vi "Do.vi"(8 "error in (no error)":errorcluster, 10 "Actor in":refnum<class "Actor.lvclass">, 11 "tt20panel_connect Msg":refnum<class "tt20panel_connect Msg.lvclass">) -> (0 "error out":errorcluster, 2 "Actor out":refnum<class "Actor.lvclass">)   [LabVIEW 2015, in "tt20panel_connect Msg.lvclass"]
doc: "This VI delivers the message to the actor by calling the appropriate method(s) on the actor."
uses:
  tt20panel_connect Msg.lvclass
  <vilib>/ActorFramework/Actor/Actor.lvclass
  tt20panel_class/tt20panel.lvclass
  tt20panel_connect Msg.lvclass/tt20panel_connect Msg.ctl
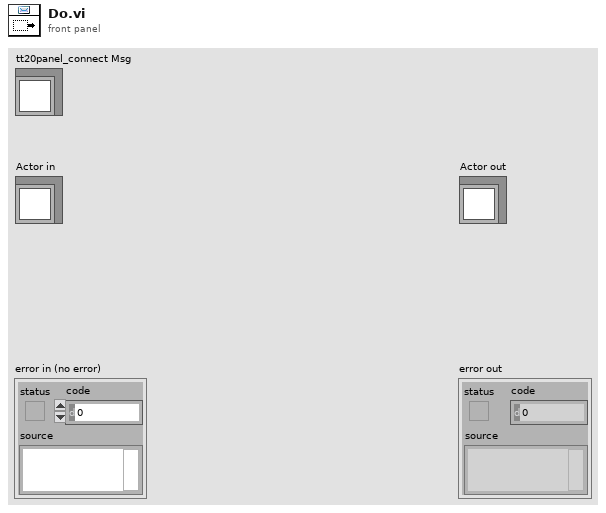
[diagram p1: front panel]
types:
  T1 = typedef "tt20_event_tdef.ctl" = cluster{"tt20_get_info":refnum<user-event>, "stream_done":refnum<user-event>, "update_status":refnum<user-event>, "update_counts":refnum<user-event>}
  T2 = typedef "tt20_hardware_info_tdef.ctl" = cluster{"model":string, "serial":string, "trigger_level":dbl[], "input_delay":i64[], "deadtime":i64[], "num_channels":u32, "status":string, "enabled":bool[], "Mode":T3, "Reference Channel":u8}
  T3 = typedef "tt20_acq_mode_tdef.ctl" = enum16{"T2", "T3"}
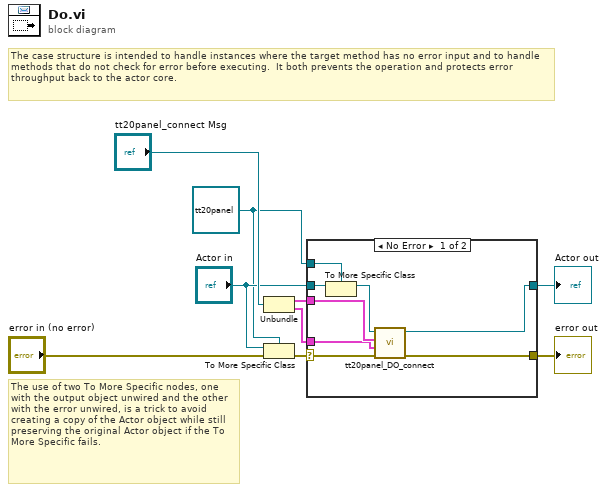
[diagram p0: block diagram]
diagram:
  w3 = refnum<class "tt20panel.lvclass"> refnum ("Actor in")
  # "The use of two To More Specific nodes, one with the output object unwired and the other with the error unwired, is a trick to avoid creating a copy of the Actor object while still preserving the original Actor object if the To More Specific fails."
  # "The case structure is intended to handle instances where the target method has no error input and to handle methods that do not check for error before executing.  It both prevents the operation and protects error throughput back to the actor core."
  n1 = Unbundle("tt20panel_connect Msg") -> (w2:T1, w1:T2)
  n2 = To More Specific Class(target class=w3, reference="Actor in", error in="error in (no error)") -> (error out=w7:errorcluster)  [unwired: 1 out]
  n3 = case shown="No Error" w7 {
    selector: w7 -> [w15 w19]
    tunnel: [w17 w19] -> w6
    tunnel: [w16 w18] -> w5
    tunnel: "Actor in" -> [w14 w18]
    tunnel: w3 -> [w13 _]
    tunnel: w2 -> [w11 _]
    tunnel: w1 -> [w10 _]
    frame No Error {
      n4 = To More Specific Class(target class=w13, reference=w14) -> (specific class reference=w12:refnum<class "tt20panel.lvclass">)  [unwired: 1 in, 1 out]
      n5 = call "tt20panel_DO_connect.vi"("error in (no error)"=w15, "tt20_settings"=w10, "tt20_events"=w11, "tt20panel in"=w12) -> ("error out"=w17:errorcluster, "tt20panel out"=w16:refnum<class "tt20panel.lvclass">)  [unwired: 6 in]
    }
    frame Error {
      # "If type check fails, pass the original object out again."
    }
  }
  "error out" <- w6
  "Actor out" <- w5
